vi "get_single_acq.vi"(8 "error in (no error)":errorcluster, 11 "Glaz-I in":refnum<class "Glaz.lvclass">) -> (0 "error out":errorcluster, 1 "wavelengths":dbl[](array[numeric]), 2 "intensity":dbl[][][](array[numeric]), 3 "Glaz-I out":refnum<class "Glaz.lvclass">, 4 "trig channel 2":bool[](array[boolean]), 6 "trig channel 1":bool[](array[boolean]))   [LabVIEW 2019, in "Glaz.lvclass"]
uses:
  Glaz.lvclass
  _cameraBase/_cameraBase.lvclass
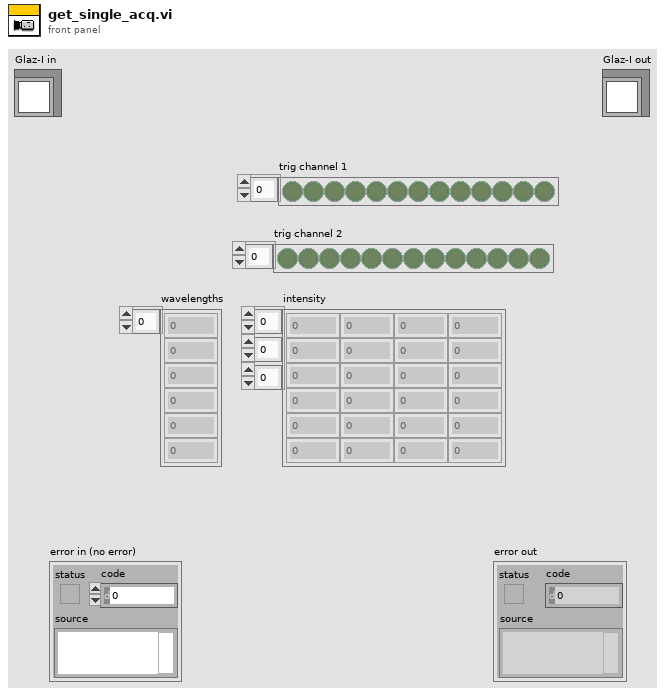
[diagram p1: front panel]
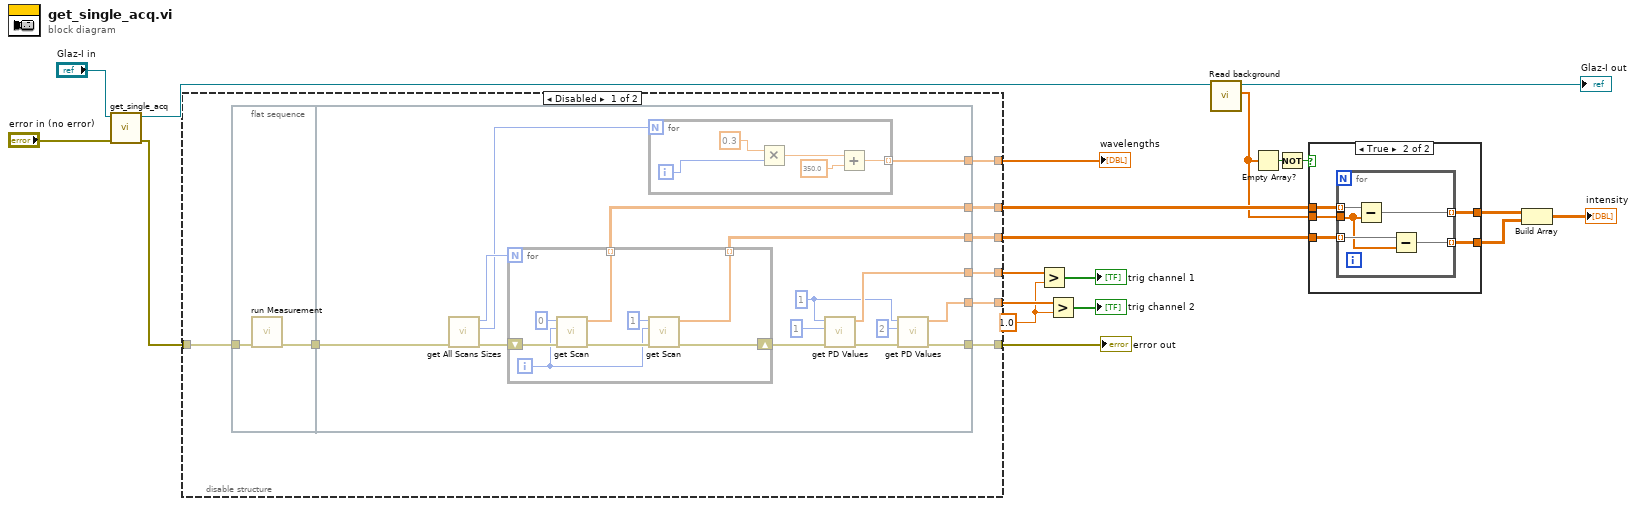
[diagram p0: block diagram]
diagram:
  w2 = 1.0
  n1 = call-parent "get_single_acq.vi"("error in (no error)"="error in (no error)", "_cameraBase in"="Glaz-I in") -> ("error out"=w18:errorcluster, "_cameraBase out"=w13:refnum<class "Glaz.lvclass">)  [unwired: 4 in, 4 out]
  n2 = disable-structure shown="Disabled" {
    disable-tunnel: w18 -> [w27 _]
    disable-tunnel: [w26 _] -> w17
    disable-tunnel: [w25 _] -> w16
    disable-tunnel: [w24 _] -> w15
    disable-tunnel: [w23 _] -> w11
    disable-tunnel: [w22 _] -> w10
    disable-tunnel: [w21 _] -> w3
    frame Disabled {
      n3 = flat-sequence {
        tunnel: [w30] -> w28
        tunnel: w27 -> [w29]
        tunnel: w28 -> [w45]
        tunnel: [w34] -> w26
        tunnel: [w41] -> w25
        tunnel: [w39] -> w24
        tunnel: [w38] -> w23
        tunnel: [w37] -> w22
        tunnel: [w31] -> w21
        frame #0 {
          n4 = call <userlib>:"run Measurement.vi"("error in (no error)"=w29) -> ("error out"=w30:errorcluster)  [unwired: 9 in, 1 out]
        }
        frame #1 {
          w33 = 1 ("pdNumber")
          n5 = call <userlib>:"get All Scans Sizes.vi"("error in (no error)"=w45) -> ("error out"=w43:errorcluster, "coloumnCount"=w42:i32, "rowCount"=w44:i32)  [unwired: 7 in, 1 out]
          n6 = for {
            N: w44 -> [_]
            shift-right: [w53] -> w40
            shift-left: w43 -> [w58]
            tunnel: [w51] -> w37 mode=indexing
            tunnel: [w52] -> w38 mode=indexing
            i -> [w54]
            n7 = call <userlib>:"get Scan.vi"("error in (no error)"=w58, "scanIndex"=w54, "calculationIndex"=0) -> ("error out"=w55:errorcluster, "values"=w52:dbl[])  [unwired: 6 in, 1 out]
            n8 = call <userlib>:"get Scan.vi"("error in (no error)"=w55, "scanIndex"=w54, "calculationIndex"=1) -> ("error out"=w53:errorcluster, "values"=w51:dbl[])  [unwired: 6 in, 1 out]
          }
          n9 = for {
            N: w42 -> [_]
            tunnel: [w46] -> w41 mode=indexing
            i -> [w50]
            n10 = Multiply(x=0.3, y=w50) -> (x*y=w48:dbl)
            n11 = Add(x=w48, y=350.0) -> (x+y=w46:dbl)
          }
          n12 = call <userlib>:"get PD Values.vi"("error in (no error)"=w40, "pdChannel"=1, "pdNumber"=w33) -> ("error out"=w35:errorcluster, "values"=w39:dbl[])  [unwired: 5 in, 1 out]
          n13 = call <userlib>:"get PD Values.vi"("error in (no error)"=w35, "pdChannel"=2, "pdNumber"=w33) -> ("error out"=w34:errorcluster, "values"=w31:dbl[])  [unwired: 5 in, 1 out]
        }
      }
    }
    frame Enabled {
    }
  }
  "error out" <- w17
  "wavelengths" <- w16
  n14 = Greater?(x=w15, y=w2) -> (0:→"trig channel 1":bool[])
  n15 = Greater?(x=w3, y=w2) -> (0:→"trig channel 2":bool[])
  n16 = call-dynamic "Read background.vi"("_cameraBase in"=w13) -> ("background"=w8:dbl[], "_cameraBase out"=→"Glaz-I out":refnum<class "Glaz.lvclass">)  [unwired: 8 in, 1 out]
  n17 = Empty Array?(array=w8) -> (empty?=w9:bool)
  n18 = Not(x=w9) -> (.not. x?=w7:bool)
  n19 = case shown="True" w7 {
    tunnel: w11 -> [w60 w65]
    tunnel: w8 -> [_ w64]
    tunnel: w10 -> [w59 w63]
    tunnel: [w60 w62] -> w6
    tunnel: [w59 w61] -> w5
    frame False {
    }
    frame True {
      n20 = for {
        tunnel: w65 -> [w70] mode=indexing
        tunnel: w64 -> [w68]
        tunnel: w63 -> [w69] mode=indexing
        tunnel: [w67] -> w61 mode=indexing
        tunnel: [w66] -> w62 mode=indexing
        n21 = Subtract(x=w70, y=w68) -> (x-y=w66:dbl[])
        n22 = Subtract(x=w69, y=w68) -> (x-y=w67:dbl[])
      }
    }
  }
  n23 = Build Array(w6, w5) -> (→"intensity":dbl[][][])
